vi "MainGui-ReasemblyDone.vi"(8 "error in (no error)":errorcluster, 10 "PLCEcho":T1) -> (0 "error out":errorcluster)   [LabVIEW 2016]
uses:
  Drivers/PLC/PLC.CheckStatusReassembly.ctl
  MainGui.Action.ctl
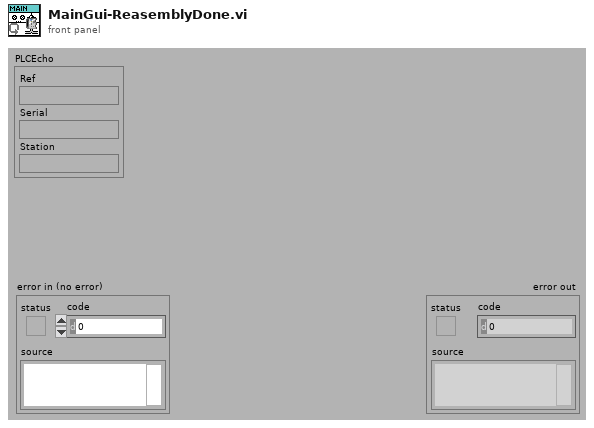
[diagram p1: front panel]
types:
  T1 = typedef "PLC.CheckStatusReassembly.ctl" = cluster{"Ref":string, "Serial":string, "Station":string}
  T2 = typedef "MainGui.Action.ctl" = enum32{"idle", "constructor", "destructor", "--- MainGui ---", "Gui.Translate", "Error.Update", "Error.Confirm", "TopBar.Update", "Buttons.Update", "StatusMsg.Update", "StatusTable.Update", "LogsTable.Update", "PLCReasemblyDone"}
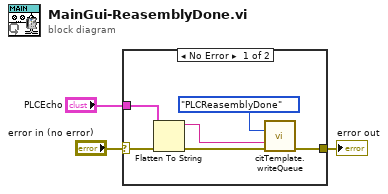
[diagram p0: block diagram]
diagram:
  n1 = case shown="No Error" "error in (no error)" {
    selector: "error in (no error)" -> [w7 w10]
    tunnel: [w9 w10] -> w2
    tunnel: "PLCEcho" -> [w5 _]
    frame No Error {
      n2 = Flatten To String(anything=w5, error in (no error)=w7) -> (data string=w4:string, error out=w6:errorcluster)  [unwired: 2 in, 1 out]
      n3 = call "citTemplate.writeQueue.vi"("event in (if not connected:all statemachine with data event)"=MainGui.Action."PLCReasemblyDone" ("Action"), "data in"=w4, "error in (no error)"=w6) -> ("error out"=w9:errorcluster)  [unwired: 12 in]
    }
    frame Error {
    }
  }
  "error out" <- w2
